vi "tareaDaq.vi"() -> ()   [LabVIEW 2011]
panel:
  in  "Boolean 2":bool
  out "Boolean":bool
  in  "stop":bool
  out "Nivel Max":bool
  out "Nivel Medio":bool
  in  "Knob":i32(knob) scale=0.0..5.0
  out "Tank":dbl(slide) scale=0.0..100.0
  # "El programa deberá de funcionar\nhasta que se presione el boton \nde detener.\nel led se debe de encender usando \nel boolean 2. en la pc y en a protox\nlos niveles max y min se tiene que \nenceder en la pc y el la protox.\n\nel tanque se llena usando el knob \nque es una señal analogica,\n1 equivale a 20.\n\nmedio es 50 y max es 80"
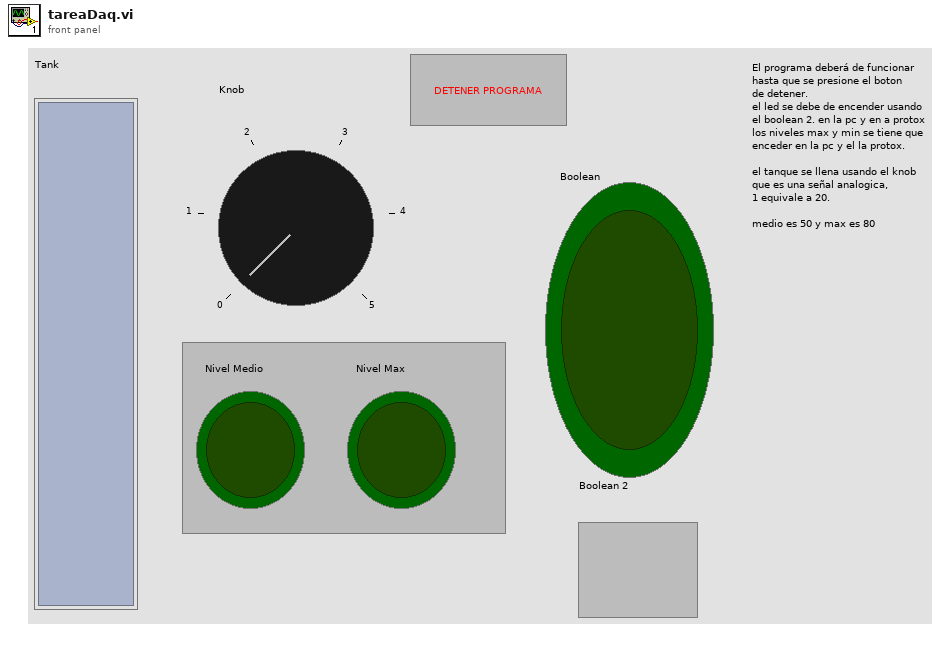
[diagram p1: front panel]
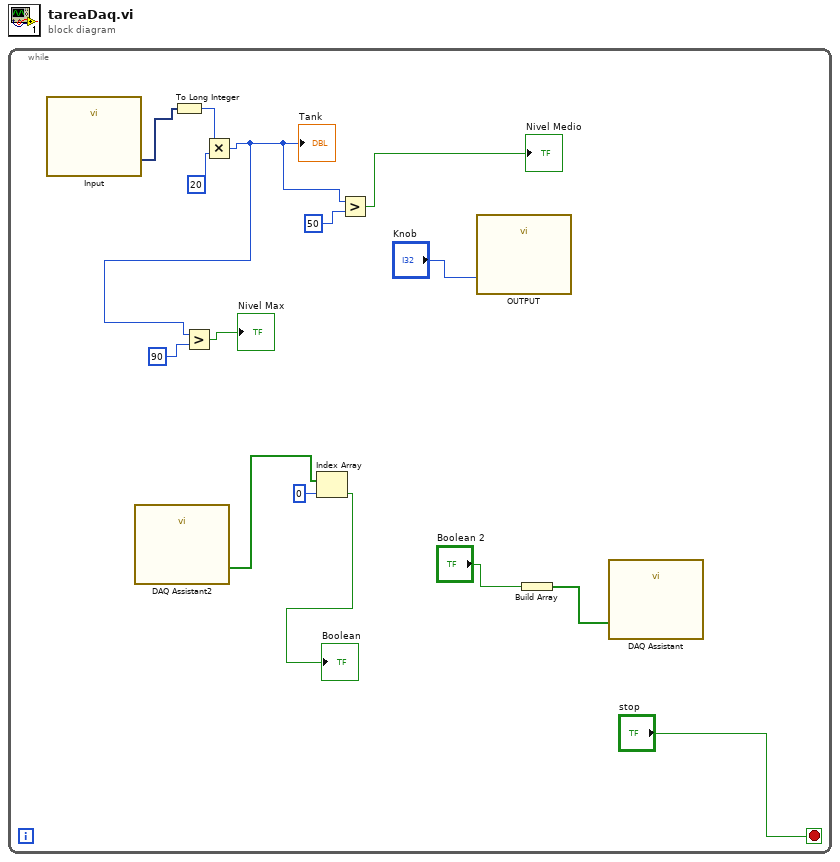
[diagram p0: block diagram]
diagram:
  n1 = while {
    stop <- "stop" stop-if-true
    n2 = call "Input"() -> ("data"=w13:dynamicdata)  [unwired: 17 in, 2 out]
    n3 = call "DAQ Assistant2"() -> ("data"=w2:bool[])  [unwired: 17 in, 2 out]
    n4 = To Long Integer(number=w13) -> (32bit integer=w12:i32)
    n5 = Multiply(x=w12, y=20) -> (x*y=w6:i32)
    "Tank" <- w6
    n6 = Greater?(x=w6, y=90) -> (0:→"Nivel Max":bool)
    n7 = Index Array "Index Array"(array=w2, index=0) -> (element=→"Boolean":bool)
    n8 = Greater?(x=w6, y=50) -> (0:→"Nivel Medio":bool)
    n9 = call "OUTPUT"("data"="Knob") -> ()  [unwired: 17 in, 2 out]
    n10 = Build Array "Build Array"("Boolean 2") -> (w4:bool[])
    n11 = call "DAQ Assistant"("data"=w4) -> ()  [unwired: 17 in, 2 out]
  }
